vi "AIT 664 - Create RT FIFOs.vi"(0 "input cluster":T1, 5 "FIFO Index Queues":T2, 11 "error in (no error)":errorcluster) -> (4 "output cluster":T1, 15 "error out":errorcluster)   [LabVIEW 2013, in "AIT 664 Custom Device.lvlib"]
doc: "Create the RT FIFOs to move data between the pcl and the async loops and the hardware in/out buffers."
uses:
  AIT 664 Custom Device.lvlib
  RT Controls/FIFO Index Queues.ctl
  RT Controls/FIFO.ctl
  RT Controls/Data Ref FGV Command.ctl
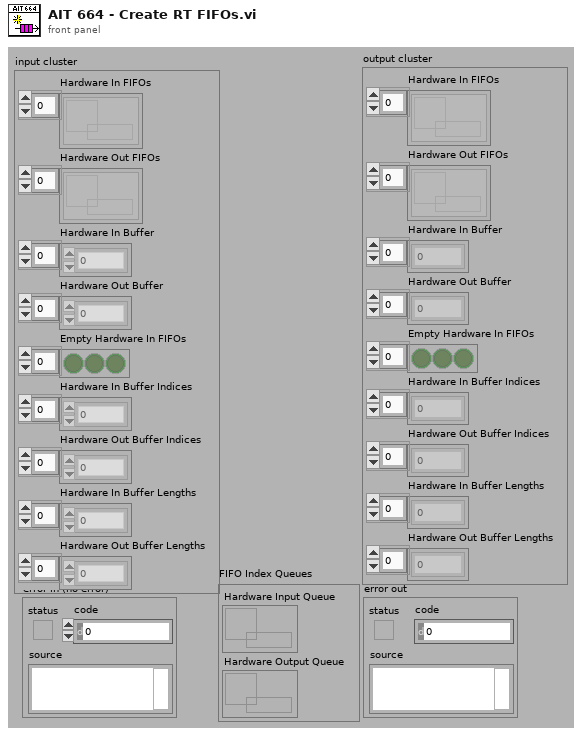
[diagram p1: front panel]
types:
  T1 = typedef "AIT 664 Custom Device.lvlib/FIFO.ctl" = cluster{"Hardware In FIFOs":refnum<k33>[], "Hardware Out FIFOs":refnum<k33>[], "Hardware In Buffer":dbl[], "Hardware Out Buffer":dbl[], "Empty Hardware In FIFOs":bool[], "Hardware In Buffer Indices":i32[], "Hardware Out Buffer Indices":i32[], "Hardware In Buffer Lengths":i32[], "Hardware Out Buffer Lengths":i32[]}
  T2 = typedef "AIT 664 Custom Device.lvlib/FIFO Index Queues.ctl" = cluster{"Hardware Input Queue":refnum<queue>, "Hardware Output Queue":refnum<queue>}
  T3 = typedef "AIT 664 Custom Device.lvlib/Data Ref FGV Command.ctl" = enum16{"Intialize", "Get", "Update"}
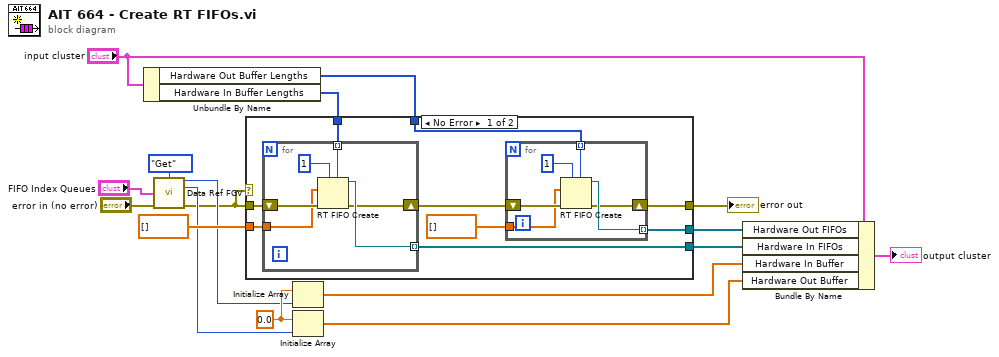
[diagram p0: block diagram]
diagram:
  w12 = 0.0
  n1 = Unbundle By Name("input cluster") -> ("Hardware Out Buffer Lengths"=w6:i32[], "Hardware In Buffer Lengths"=w10:i32[])
  n2 = call "Data Ref FGV.vi"("Action"=Data_Ref_FGV_Command."Get" ("Command"), "FIFO Index Queues"="FIFO Index Queues", "error in (no error)"="error in (no error)") -> ("Hardware Input FIFO Index"=w4:i32, "Hardware Output FIFO Index"=w3:i32, "error out"=w1:errorcluster)  [unwired: 10 in]
  n3 = case shown="No Error" w1 {
    tunnel: w1 -> [w26 w39]
    tunnel: dbl[] [] -> [w25 _]
    tunnel: [w21 w39] -> w11
    tunnel: w10 -> [w24 _]
    tunnel: [w23 _] -> w9
    tunnel: w6 -> [w20 _]
    tunnel: [w19 _] -> w2
    frame No Error {
      n4 = for {
        tunnel: [w37] -> w23 mode=indexing
        tunnel: w25 -> [w35]
        tunnel: w24 -> [w34] mode=indexing
        shift-right: [w33] -> w22
        shift-left: w26 -> [w38]
        n5 = RT FIFO Create(1:w35, 3:w38, 4:u32 1 ("size (10)"), 6:w34) -> (8:w37:refnum<k33>, 11:w33:errorcluster)  [unwired: 4 in, 1 out]
      }
      n6 = for {
        tunnel: [w31] -> w19 mode=indexing
        tunnel: dbl[] [] -> [w29]
        tunnel: w20 -> [w28] mode=indexing
        shift-right: [w27] -> w21
        shift-left: w22 -> [w32]
        n7 = RT FIFO Create(1:w29, 3:w32, 4:u32 1 ("size (10)"), 6:w28) -> (8:w31:refnum<k33>, 11:w27:errorcluster)  [unwired: 4 in, 1 out]
      }
    }
    frame Error {
    }
  }
  "error out" <- w11
  n8 = Initialize Array(w12, w4) -> (w8:dbl[])
  n9 = Initialize Array(w12, w3) -> (w7:dbl[])
  n10 = Bundle By Name(cluster="input cluster", "Hardware Out FIFOs"=w2, "Hardware In FIFOs"=w9, "Hardware In Buffer"=w8, "Hardware Out Buffer"=w7) -> (→"output cluster":T1)
